vi "Parse Main Body.vi"(8 "Error In":errorcluster, 11 "Main Body":string[](array[string])) -> (0 "Error Out":errorcluster, 3 "Provisional Line Items":T1[](array[typedef]) {"PriceIncDiscount (£)" format="%.2g"; "Discount(£)" format="%.2g"})   [LabVIEW 2018, in "Receipt Parsing.lvlib"]
uses:
  Receipt Parsing.lvlib
  ReceiptItemInfo.ctl
  database/Items--cluster.ctl
  database/Database.lvlib
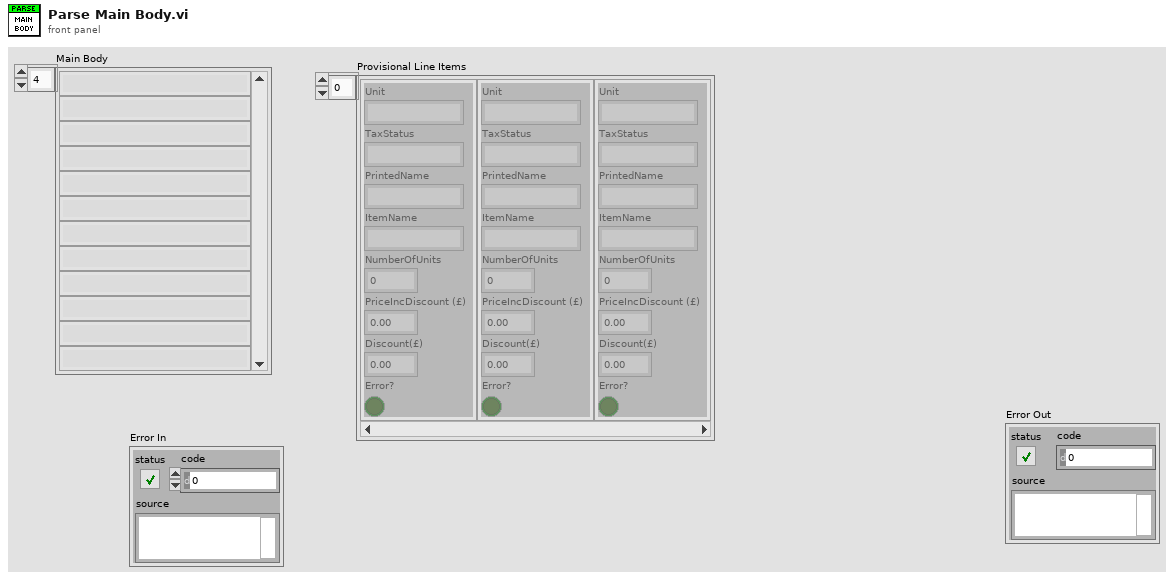
[diagram p1: front panel]
types:
  T1 = typedef "Receipt Parsing.lvlib/ReceiptItemInfo.ctl" = cluster{"Unit":string, "TaxStatus":string, "PrintedName":string, "ItemName":string, "NumberOfUnits":dbl, "PriceIncDiscount (£)":dbl, "Discount(£)":dbl, "Error?":bool}
  T2 = typedef "Database.lvlib/Items--cluster.ctl" = cluster{"ItemName":string, "FriendlyName":string, "IsFood":bool, "IsVeg":bool, "IsFavourite":bool}
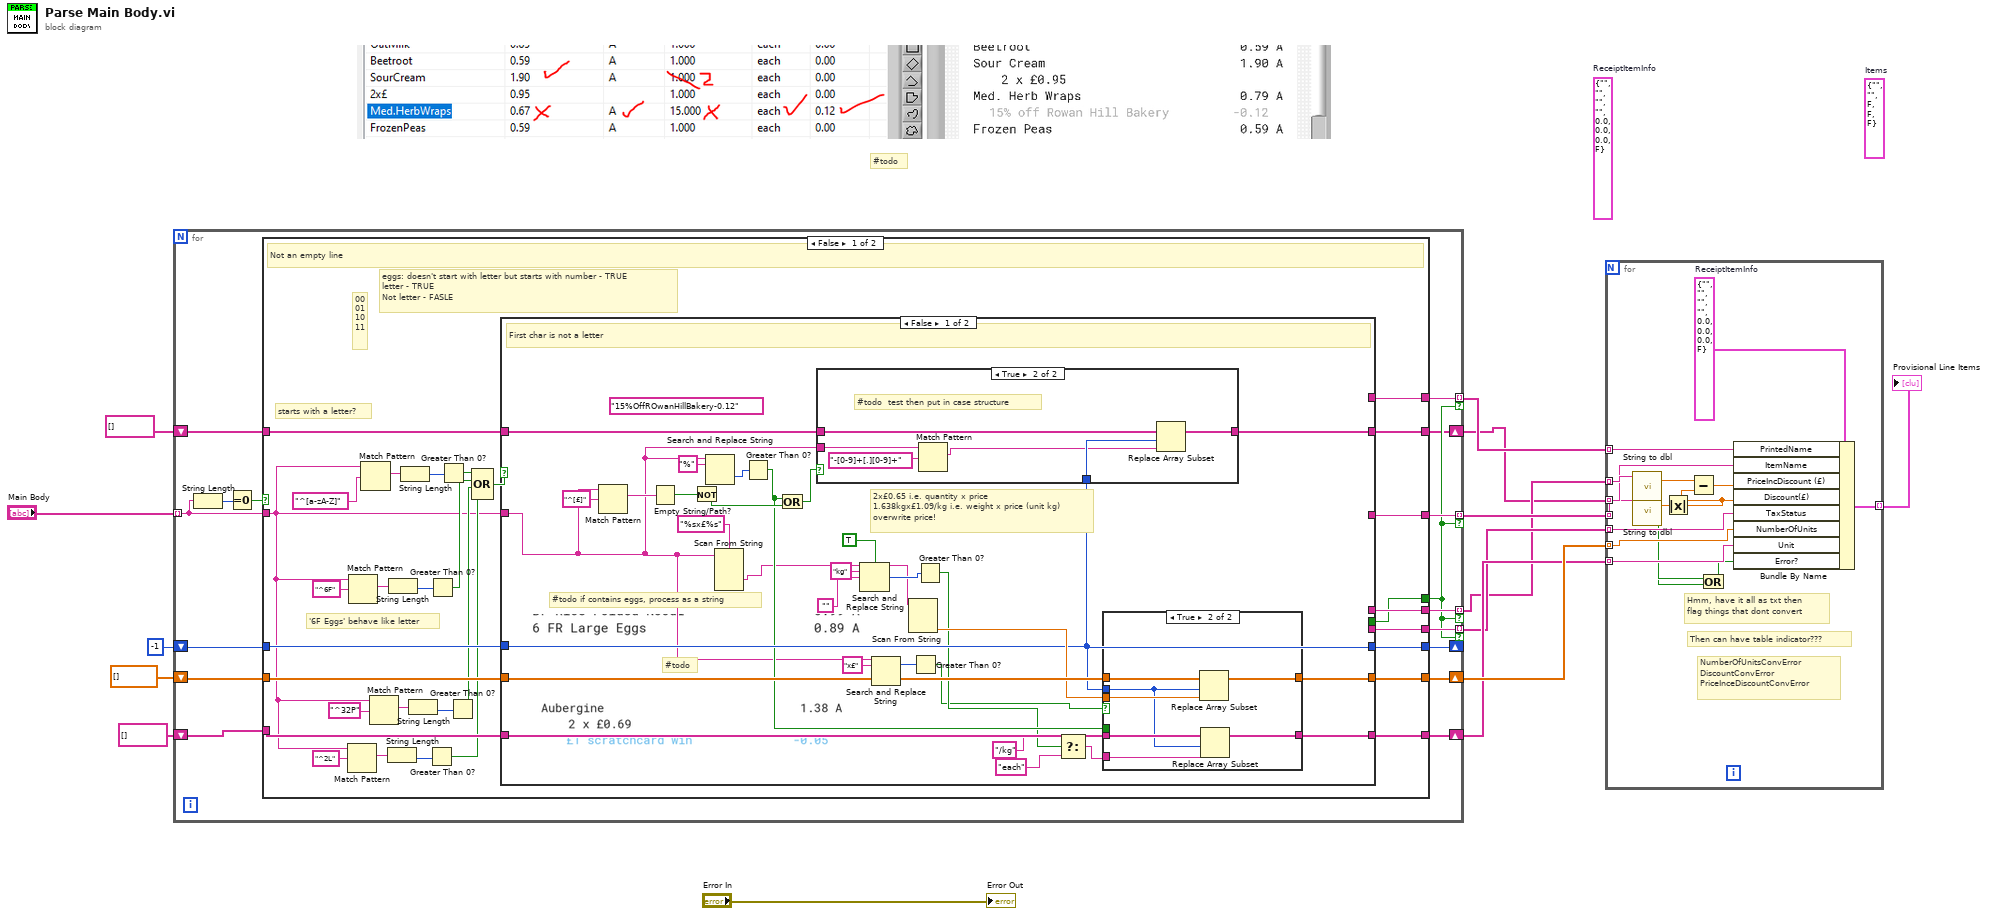
[diagram p0: block diagram]
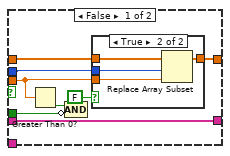
[diagram p3: hidden frame]
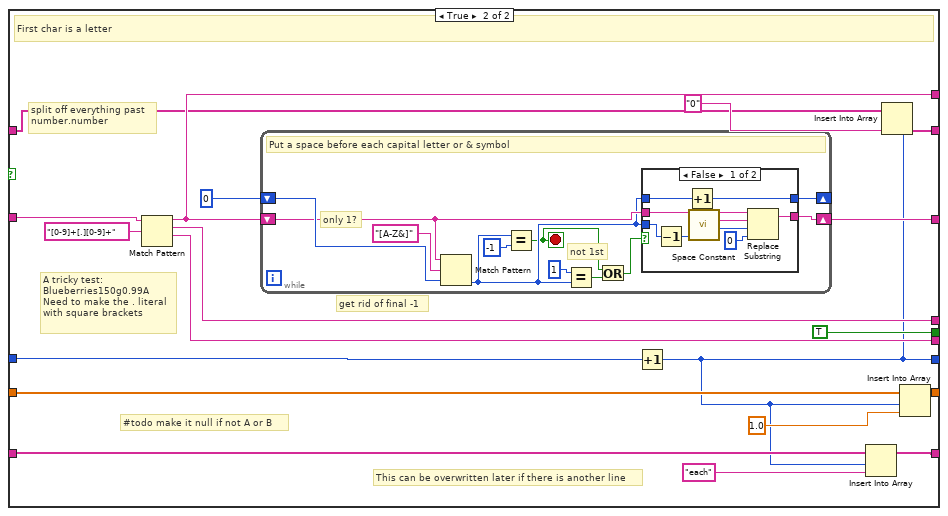
[diagram p5: hidden frame]
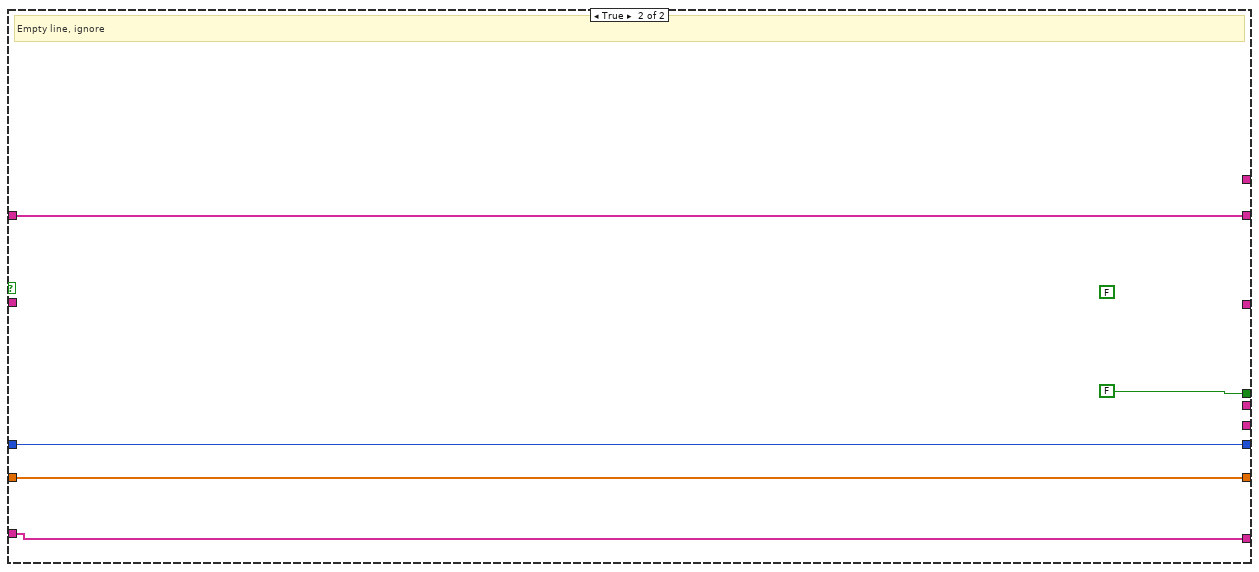
[diagram p7: hidden frame]
diagram:
  (unwired) T2 {"ItemName"="", "FriendlyName"="", "IsFood"=FALSE, "IsVeg"=FALSE, "IsFavourite"=FALSE}  # Items
  (unwired) T1 {"Unit"="", "TaxStatus"="", "PrintedName"="", "ItemName"="", "NumberOfUnits"=0.0, "PriceIncDiscount (£)"=0.0, "Discount(£)"=0.0, "Error?"=FALSE}  # ReceiptItemInfo
  # "#todo"
  n1 = for {
    tunnel: "Main Body" -> [w28] mode=indexing
    tunnel: [w30] -> w7 mode=indexing if=w17
    tunnel: [w29] -> w3 mode=indexing if=w17
    tunnel: [w25] -> w8 mode=indexing if=w17
    tunnel: [w24] -> w4 mode=indexing if=w17
    shift-right: [w23] -> w6
    shift-left: dbl[] [] -> [w22]
    shift-right: [w20] -> _
    shift-left: -1 -> [w21]
    shift-right: [w19] -> w5
    shift-left: string[] [] -> [w18]
    shift-right: [w16] -> w2
    shift-left: string[] [] -> [w15]
    n2 = String Length(string=w28) -> (length=w27:i32)
    n3 = Equal To 0?(x=w27) -> (x = 0?=w26:bool)
    n4 = case shown="False" w26 {
      tunnel: [w61 _] -> w30
      tunnel: [w60 _] -> w29
      tunnel: w28 -> [w31 _]
      tunnel: [w56 FALSE] -> w17
      tunnel: [w55 _] -> w25
      tunnel: [w54 _] -> w24
      tunnel: [w51 w163] -> w23
      tunnel: w22 -> [w50 w163]
      tunnel: w21 -> [w52 w162]
      tunnel: [w53 w162] -> w20
      tunnel: [w49 w161] -> w19
      tunnel: w18 -> [w48 w161]
      tunnel: [w47 w160] -> w16
      tunnel: w15 -> [w46 w160]
      frame False {
        # "eggs: doesn't start with letter but starts with number - TRUE\nletter - TRUE\nNot letter - FASLE"
        # "00\n01\n10\n11"
        # "'6F Eggs' behave like letter"
        # "starts with a letter?"
        # "Not an empty line"
        n5 = Match Pattern(string=w31, regular expression="^2L") -> (match substring=w34:string)  [unwired: 1 in, 3 out]
        n6 = Match Pattern(string=w31, regular expression="^6F") -> (match substring=w44:string)  [unwired: 1 in, 3 out]
        n7 = Match Pattern(string=w31, regular expression="^[a-zA-Z]") -> (match substring=w57:string)  [unwired: 1 in, 3 out]
        n8 = Match Pattern(string=w31, regular expression="^32P") -> (match substring=w38:string)  [unwired: 1 in, 3 out]
        n9 = String Length(string=w34) -> (length=w33:i32)
        n10 = String Length(string=w44) -> (length=w41:i32)
        n11 = String Length(string=w57) -> (length=w59:i32)
        n12 = String Length(string=w38) -> (length=w37:i32)
        n13 = Greater Than 0?(x=w33) -> (x > 0?=w32:bool)
        n14 = Greater Than 0?(x=w41) -> (x > 0?=w40:bool)
        n15 = Greater Than 0?(x=w59) -> (x > 0?=w43:bool)
        n16 = Greater Than 0?(x=w37) -> (x > 0?=w36:bool)
        n17 = Compound Arithmetic op=OR(w43, w40, w36, w32) -> (w42:bool)
        n18 = case shown="False" w42 {
          tunnel: w31 -> [w64 w136]
          tunnel: [_ w137] -> w61
          tunnel: [_ w134] -> w60
          tunnel: [_ TRUE] -> w56
          tunnel: [_ w132] -> w55
          tunnel: [_ w131] -> w54
          tunnel: [w77 w120] -> w53
          tunnel: w52 -> [w77 w130]
          tunnel: [w85 w129] -> w51
          tunnel: w50 -> [w86 w128]
          tunnel: [w83 w126] -> w49
          tunnel: w48 -> [w82 w125]
          tunnel: [w79 w123] -> w47
          tunnel: w46 -> [w78 w121]
          frame False {
            (unwired) "15%OffROwanHillBakery-0.12"
            # "#todo"
            # "#todo if contains eggs, process as a string"
            # "2x£0.65 i.e. quantity x price\n1.638kgx£1.09/kg i.e. weight x price (unit kg)\noverwrite price!"
            # "First char is not a letter"
            n19 = Match Pattern(string=w64, regular expression="^[£]") -> (match substring=w75:string)  [unwired: 1 in, 3 out]
            n20 = Empty String/Path?(string/path=w75) -> (empty?=w74:bool)
            n21 = Not(x=w74) -> (.not. x?=w73:bool)
            n22 = Search and Replace String(input string=w64, search string="%") -> (offset past replacement=w80:i32)  [unwired: 6 in, 3 out]
            n23 = Scan From String(format string="%sx£%s", input string=w64) -> (output 1=w66:string)  [unwired: 5 in, 3 out]
            n24 = Greater Than 0?(x=w80) -> (x > 0?=w71:bool)
            n25 = Or(x=w71, y=w73) -> (x .or. y?=w72:bool)
            n26 = case shown="True" w72 {
              tunnel: w64 -> [_ w98]
              tunnel: [w93 w97] -> w79
              tunnel: w78 -> [w93 w96]
              tunnel: w77 -> [_ w95]
              frame False {
              }
              frame True {
                # "#todo  test then put in case structure"
                n27 = Match Pattern(string=w98, regular expression="-[0-9]+[.][0-9]+") -> (match substring=w94:string)  [unwired: 1 in, 3 out]
                n28 = Replace Array Subset(array=w96, new element=w94, index=w95) -> (w97:string[])
              }
            }
            n29 = Search and Replace String(case sensitive?=TRUE ("ignore case? (F)"), input string=w66, search string="kg", replace string="") -> (result string=w87:string, number of replacements=w89:i32)  [unwired: 4 in, 2 out]
            n30 = Search and Replace String(input string=w64, search string="x£") -> (number of replacements=w63:i32)  [unwired: 6 in, 3 out]
            n31 = Scan From String(input string=w87) -> (output 1=w84:dbl)  [unwired: 4 in, 3 out]
            n32 = Greater Than 0?(x=w63) -> (x > 0?=w62:bool)
            n33 = Greater Than 0?(x=w89) -> (x > 0?=w69:bool)
            n34 = Select(t="/kg" ("search string"), s=w69, f="each") -> (s? t:f=w70:string)
            n35 = case shown="True" w62 {
              tunnel: w86 -> [w106 w119]
              tunnel: [w105 w118] -> w85
              tunnel: w84 -> [w103 w117]
              tunnel: w77 -> [w104 w114]
              tunnel: [w107 w116] -> w83
              tunnel: w82 -> [w107 w115]
              tunnel: w71 -> [w101 _]
              tunnel: w70 -> [_ w113]
              frame False {
                n36 = Greater Than 0?(x=w103) -> (x > 0?=w102:bool)
                n37 = Compound Arithmetic op=AND(w102, invert w101) -> ()  [unwired: 1 out]
                n38 = case shown="True" FALSE {
                  tunnel: w106 -> [w108 w112]
                  tunnel: [w108 w111] -> w105
                  tunnel: w104 -> [_ w110]
                  tunnel: w103 -> [_ w109]
                  frame False {
                  }
                  frame True {
                    n39 = Replace Array Subset(array=w112, new element=w109, index=w110) -> (w111:dbl[])
                  }
                }
              }
              frame True {
                n40 = Replace Array Subset(array=w119, new element=w117, index=w114) -> (w118:dbl[])
                n41 = Replace Array Subset(array=w115, new element=w113, index=w114) -> (w116:string[])
              }
            }
          }
          frame True {
            # "A tricky test:\nBlueberries150g0.99A\nNeed to make the . literal\nwith square brackets"
            # "This can be overwritten later if there is another line"
            # "#todo make it null if not A or B"
            # "split off everything past\nnumber.number"
            # "get rid of final -1"
            # "First char is a letter"
            n42 = Match Pattern(string=w136, regular expression="[0-9]+[.][0-9]+") -> (before substring=w132:string, match substring=w134:string, after substring=w131:string)  [unwired: 1 in, 1 out]
            n43 = while {
              shift-right: [w144] -> _
              shift-left: 0 ("offset past match") -> [w147]
              shift-right: [w146] -> w137
              shift-left: w132 -> [w145]
              stop <- w140 stop-if-true
              # "not 1st"
              # "only 1?"
              # "Put a space before each capital letter or & symbol"
              n44 = Match Pattern(string=w145, regular expression="[A-Z&]", offset (0)=w147) -> (offset past match=w142:i32)  [unwired: 3 out]
              n45 = Equal?(x=w142, y=-1) -> (x = y?=w140:bool)
              n46 = Equal?(x=1, y=w142) -> (x = y?=w143:bool)
              n47 = Or(x=w140, y=w143) -> (x .or. y?=w141:bool)
              n48 = case shown="False" w141 {
                tunnel: w142 -> [w154 _]
                tunnel: [w156 w159] -> w146
                tunnel: w145 -> [w155 w159]
                tunnel: w142 -> [w151 w158]
                tunnel: [w150 w158] -> w144
                frame False {
                  n49 = Decrement(x=w154) -> (x-1=w153:i32)
                  n50 = Increment(x=w151) -> (x+1=w150:i32)
                  n51 = call <vilib>:"Space Constant.vi"() -> ("String"=w157:string)
                  n52 = Replace Substring(2:0 ("length (len. of substring)"), 3:w153, 4:w157, 5:w155) -> (1:w156:string)  [unwired: 1 out]
                }
                frame True {
                }
              }
            }
            n53 = Increment(x=w130) -> (x+1=w120:i32)
            n54 = Insert Into Array(array=w125, index=w120, new element="each" ("new element/subarray")) -> (w126:string[])
            n55 = Insert Into Array(array=w121, index=w120, new element="0" ("Read String")) -> (w123:string[])
            n56 = Insert Into Array(array=w128, index=w120, new element=1.0) -> (w129:dbl[])
          }
        }
      }
      frame True {
        (unwired) FALSE
        # "Empty line, ignore"
      }
    }
  }
  n57 = for {
    tunnel: w8 -> [w179] mode=indexing
    tunnel: w7 -> [w173] mode=indexing
    tunnel: w6 -> [w178] mode=indexing
    tunnel: w5 -> [w177] mode=indexing
    tunnel: w4 -> [w176] mode=indexing
    tunnel: [w175] -> w1 mode=indexing
    tunnel: w3 -> [w174] mode=indexing
    tunnel: w2 -> [w172] mode=indexing
    w180 = T1 {"Unit"="", "TaxStatus"="", "PrintedName"="", "ItemName"="", "NumberOfUnits"=0.0, "PriceIncDiscount (£)"=0.0, "Discount(£)"=0.0, "Error?"=FALSE}  # ReceiptItemInfo
    # "Then can have table indicator???"
    # "NumberOfUnitsConvError\nDiscountConvError\nPriceInceDiscountConvError"
    # "Hmm, have it all as txt then\nflag things that dont convert"
    n58 = call "String to dbl.vi"("String"=w174) -> ("Error?"=w169:bool, "dbl"=w171:dbl)  [unwired: 9 in]
    n59 = call "String to dbl.vi"("String"=w172) -> ("Error?"=w168:bool, "dbl"=w166:dbl)  [unwired: 9 in]
    n60 = Absolute Value(x=w166) -> (abs(x)=w165:dbl)
    n61 = Subtract(x=w171, y=w165) -> (x-y=w170:dbl)
    n62 = Or(x=w169, y=w168) -> (x .or. y?=w167:bool)
    n63 = Bundle By Name(cluster=w180, "PrintedName"=w179, "ItemName"=w173, "PriceIncDiscount (£)"=w170, "Discount(£)"=w165, "TaxStatus"=w176, "NumberOfUnits"=w178, "Unit"=w177, "Error?"=w167) -> (w175:T1)
  }
  "Provisional Line Items" <- w1
  "Error Out" <- "Error In"
